vi "Read TDMS File Parameters.vi"() -> ()   [LabVIEW 2011]
panel:
  out "element 0":string
  out "element 4":string
  out "property value 4":i32
  out "property value 3":string
  out "element 3":string
  out "element 2":string
  out "property value 2":i32
  out "property value 1":i32
  out "element 1":string
  out "element":variant
  out "channel names":string[](array[string])
  out "group names":string[](array[string])
  out "property names 2":string[](array[string])
  out "property value 0":variant
  out "property values":variant[](array[variant])
  out "property names":string[](array[string])
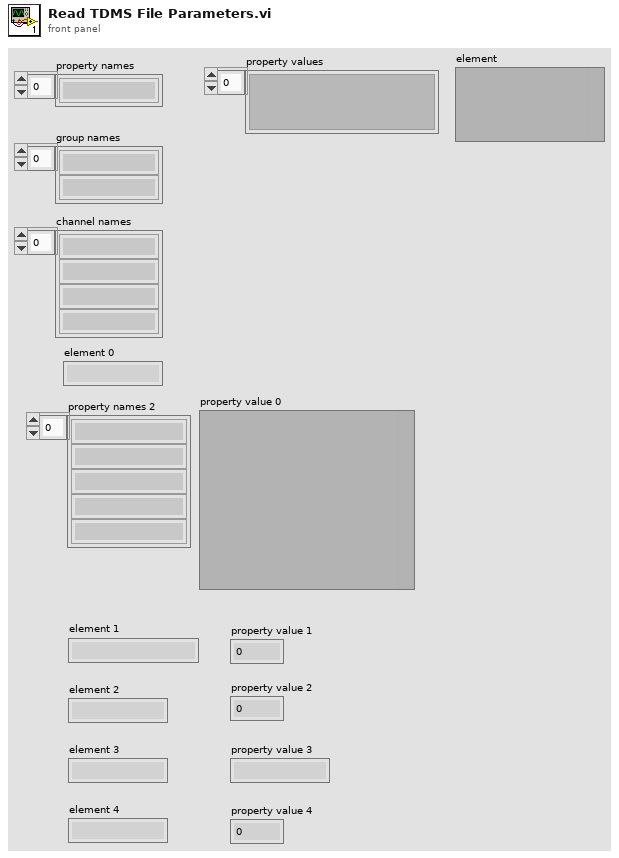
[diagram p1: front panel]
types:
  T1 = enum16{"open", "open or create", "create or replace", "create", "open (read-only)"}
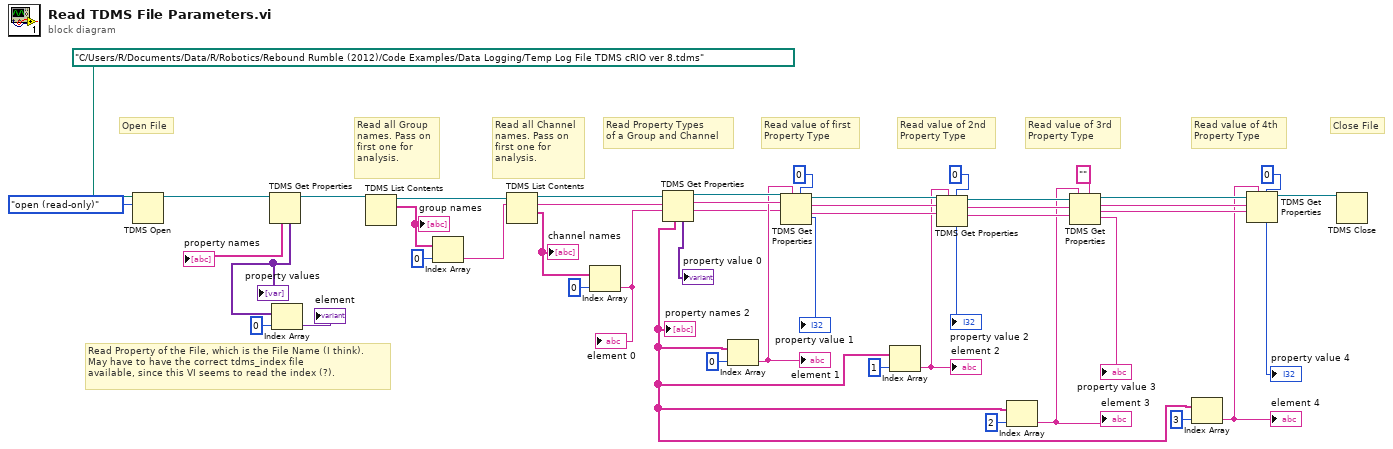
[diagram p0: block diagram]
diagram:
  # "Close File"
  # "Read value of 4th\nProperty Type"
  # "Read value of 3rd\nProperty Type"
  # "Read value of 2nd\nProperty Type"
  # "Read value of first\nProperty Type"
  # "Read Property Types \nof a Group and Channel"
  # "Read all Channel\nnames. Pass on\nfirst one for\nanalysis."
  # "Open File"
  # "Read all Group\nnames. Pass on\nfirst one for\nanalysis."
  # "Read Property of the File, which is the File Name (I think).\nMay have to have the correct tdms_index file\navailable, since this VI seems to read the index (?)."
  n1 = TDMS Open(10:T1."open (read-only)" ("operation (0:open)"), 11:path "C:/Users/R/Documents/Data/R/Robotics/Rebound Rumble (2012)/Code Examples/Data Logging/Temp Log File TDMS cRIO ver 8.tdms" ("file path")) -> (3:w47:refnum<k34>)  [unwired: 4 in, 1 out]
  n2 = TDMS Get Properties(11:w47) -> (3:w38:refnum<k34>, 4:w45:variant[], 6:→"property names":string[])  [unwired: 5 in, 3 out]
  "property values" <- w45
  n3 = Index Array(array=w45, index=0) -> (element=→"element":variant)
  n4 = TDMS List Contents(7:w38) -> (2:w41:string[], 3:w42:refnum<k34>)  [unwired: 2 in, 2 out]
  "group names" <- w41
  n5 = Index Array(array=w41, index=0) -> (element=w39:string)
  n6 = TDMS List Contents(6:w39, 7:w42) -> (1:w33:string[], 2:w36:string, 3:w37:refnum<k34>)  [unwired: 1 in, 1 out]
  "channel names" <- w33
  n7 = Index Array(array=w33, index=0) -> (element=w32:string)
  "element 0" <- w32
  n8 = TDMS Get Properties(9:w32, 10:w36, 11:w37) -> (1:w27:string, 2:w30:string, 3:w31:refnum<k34>, 4:→"property value 0":variant[], 6:w4:string[])  [unwired: 3 in, 1 out]
  "property names 2" <- w4
  n9 = Index Array(array=w4, index=0) -> (element=w28:string)
  "element 1" <- w28
  n10 = TDMS Get Properties(5:0 ("index"), 7:w28, 9:w27, 10:w30, 11:w31) -> (1:w21:string, 2:w22:string, 3:w24:refnum<k34>, 4:→"property value 1":i32)  [unwired: 1 in, 2 out]
  n11 = Index Array(array=w4, index=1) -> (element=w20:string)
  "element 2" <- w20
  n12 = TDMS Get Properties(5:0 ("index"), 7:w20, 9:w21, 10:w22, 11:w24) -> (1:w15:string, 2:w16:string, 3:w17:refnum<k34>, 4:→"property value 2":i32)  [unwired: 1 in, 2 out]
  n13 = Index Array(array=w4, index=2) -> (element=w11:string)
  "element 3" <- w11
  n14 = TDMS Get Properties(5:"", 7:w11, 9:w15, 10:w16, 11:w17) -> (1:w5:string, 2:w6:string, 3:w7:refnum<k34>, 4:→"property value 3":string)  [unwired: 1 in, 2 out]
  n15 = Index Array(array=w4, index=3) -> (element=w3:string)
  "element 4" <- w3
  n16 = TDMS Get Properties(5:0 ("index"), 7:w3, 9:w5, 10:w6, 11:w7) -> (3:w8:refnum<k34>, 4:→"property value 4":i32)  [unwired: 1 in, 4 out]
  n17 = TDMS Close(11:w8) -> ()  [unwired: 1 in, 2 out]
